vi "Utility Parse User Compensation.vi"(8 "error in (no error)":errorcluster, 11 "Input String":string) -> (0 "error out":errorcluster, 3 "Compensation":dbl)   [LabVIEW 2020, in "ChromTech MX-Class Drivers.lvlib"]
uses:
  <instrlib>/RxnRover/ChromtechNextGenDriver/ChromTech MX-Class Drivers.lvlib
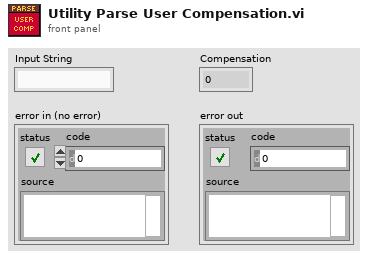
[diagram p1: front panel]
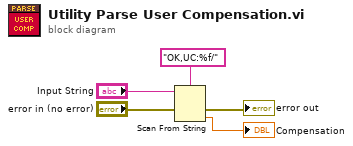
[diagram p0: block diagram]
diagram:
  n1 = Scan From String(format string="OK,UC:%f/", input string="Input String", error in="error in (no error)") -> (error out=→"error out":errorcluster, output 1=→"Compensation":dbl)  [unwired: 2 in, 2 out]
